vi "Configure Trigger Modifier [TM] Core.vi"(8 "error in (no error)":errorcluster, 10 "trigger modifier (None)":i32(ring)=1 items=["None"=1, "Auto"=2, "Auto Level"=3], 11 "CS++Scope":refnum<class "CS++Scope.lvclass">) -> (0 "error out":errorcluster, 3 "CS++Scope out":refnum<class "CS++Scope.lvclass">)   [LabVIEW 2015, in "CS++Scope.lvlib" / "CS++Scope.lvclass"]
doc: "This VI configures the trigger modifier. The trigger modifier determines the oscilloscope's behavior in the absence of the configured trigger.\n\nNote: This VI is part of the IviScopeTriggerModifier [TM] extension group."
uses:
  CS++Scope.lvclass
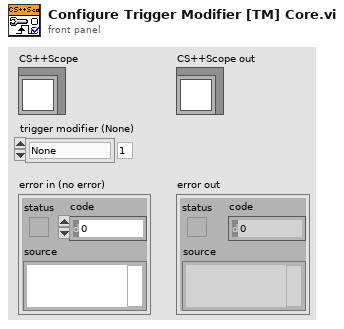
[diagram p1: front panel]
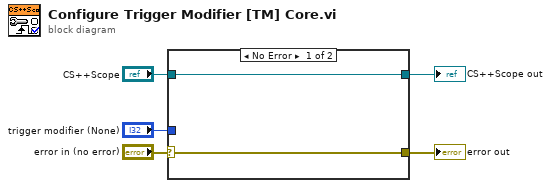
[diagram p0: block diagram]
diagram:
  n1 = case shown="No Error" "error in (no error)" {
    selector: "error in (no error)" -> [w6 w9]
    tunnel: [w6 w9] -> w4
    tunnel: [w7 w8] -> w2
    tunnel: "CS++Scope" -> [w7 w8]
    tunnel: "trigger modifier (None)" -> [_ _]
    frame No Error {
    }
    frame Error {
    }
  }
  "error out" <- w4
  "CS++Scope out" <- w2
